vi "latch variable panel controller test.vi"() -> ()   [LabVIEW 2010]
panel:
  out "Front Panel Window:State":T1(ring)
  out "Label.Text":string
  out "x+y":i16
  in  "stop":bool
  in  "OK Button":bool
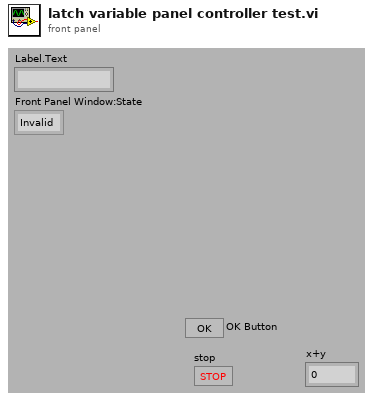
[diagram p1: front panel]
types:
  T1 = enum32{"Invalid", "Standard", "Closed", "Hidden", "Minimized", "Maximized"}
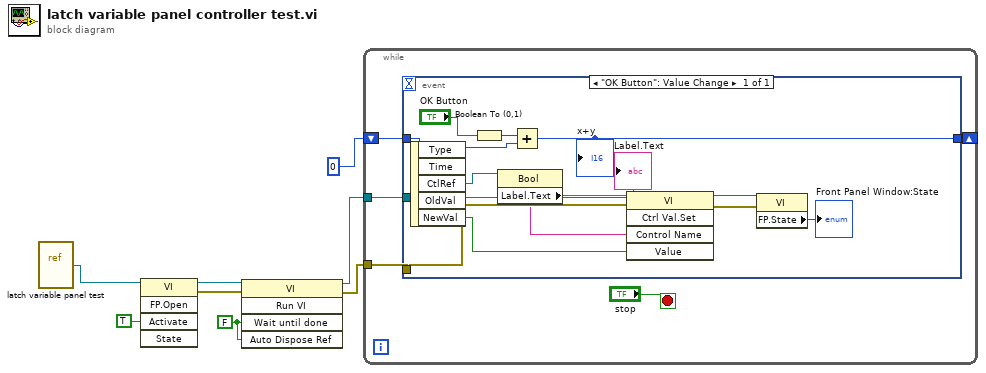
[diagram p0: block diagram]
diagram:
  w4 = FALSE ("Wait Until Done")
  n1 = vi-ref "latch variable panel test.vi"() -> (w3:refnum<vi>)
  n2 = invoke class="VI" method="FP.Open"(reference=w3, "Activate"=TRUE ("Activate?")) -> (reference out=w5:refnum<vi>, error out=w6:errorcluster)  [unwired: 3 in, 3 out]
  n3 = invoke class="VI" method="Run VI"(reference=w5, error in=w6, "Wait until done"=w4, "Auto Dispose Ref"=w4) -> (reference out=w2:refnum<vi>, error out=w1:errorcluster)  [unwired: 1 in, 3 out]
  n4 = while {
    shift-right: [w12] -> _
    shift-left: i16 0 ("Numeric") -> [w11]
    tunnel: w2 -> [w10]
    tunnel: w1 -> [w9]
    stop <- "stop" stop-if-true
    n5 = event shown="[0] \"OK Button\": Value Change" {
      selector: _ -> [_]
      dyn-events: _ -> [_]
      timeout: _ -> [_]
      tunnel: [w24] -> w12
      tunnel: w11 -> [w23]
      tunnel: w10 -> [w22]
      tunnel: w9 -> [w21]
      event "OK Button": Value Change {
        n6 = event-data() -> ("CtlRef"=w19:refnum<vi>, "NewVal"=w18:bool)  [unwired: 1 in, 3 out]
        n7 = Boolean To (0,1)(Boolean="OK Button") -> (0, 1=w25:i16)
        n8 = property class="Bool"(reference=w19) -> ("Label.Text"=w20:string)  [unwired: 1 in, 2 out]
        "Label.Text" <- w20
        n9 = Add(x=w25, y=w23) -> (x+y=w24:i16)
        "x+y" <- w24
        n10 = invoke class="VI" method="Ctrl Val.Set"(reference=w22, error in=w21, "Control Name"=w20, "Value"=w18) -> (reference out=w16:refnum<vi>, error out=w15:errorcluster)  [unwired: 1 in, 3 out]
        n11 = property class="VI"(reference=w16, error in=w15) -> ("FP.State"=→"Front Panel Window:State":T1)  [unwired: 2 out]
      }
    }
  }
